vi "XY Graph.vi"() -> ()   [LabVIEW 2023]
uses:
  <vilib>/Utility/file.llb/Read Delimited Spreadsheet (DBL).vi
panel:
  out "XY Graph 3":cluster{dbl[], "all rows":dbl[]}[](graph)
  out "y":dbl[](array[numeric])
  out "x":dbl[](array[numeric])=[1.0, 2.0, 3.0, 4.0, 5.0, 6.0]
  out "XY Graph 2":cluster{dbl[], "all rows":dbl[]}(graph)
  out "y":dbl[](array[numeric])
  out "y":dbl[](array[numeric])
  in  "file path (dialog if empty)":path
  out "XY Graph":cluster{"Y":dbl[], "Y":dbl[]}[](graph)
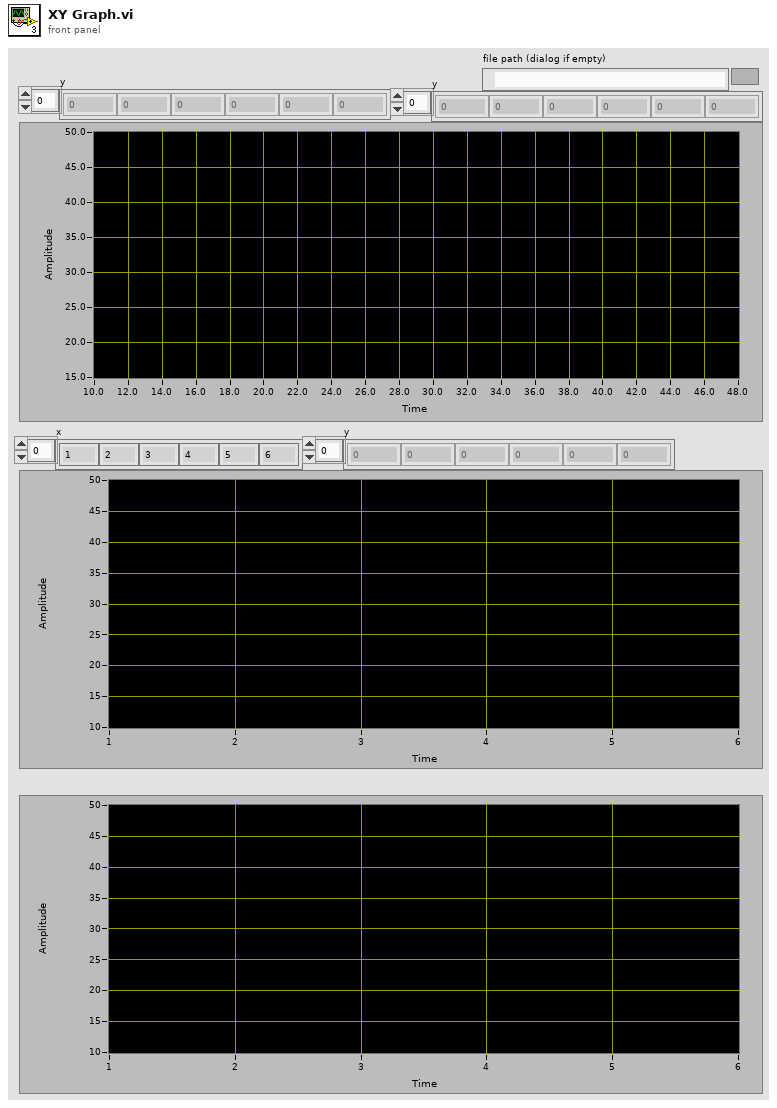
[diagram p1: front panel]
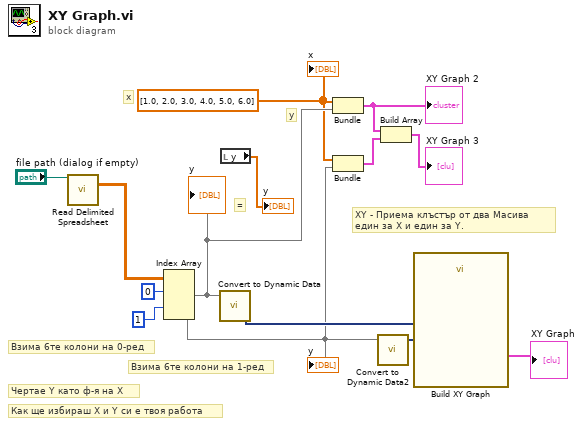
[diagram p0: block diagram]
diagram:
  w6 = dbl[] [1.0, 2.0, 3.0, 4.0, 5.0, 6.0]
  # "Как ще избираш X и Y си е твоя работа"
  # "Чертае Y като ф-я на Х"
  # "XY - Приема клъстър от два Масива\nедин за Х и един за Y."
  # "Взима 6те колони на 1-ред"
  # "Взима 6те колони на 0-ред"
  # "="
  # "y"
  # "x"
  n1 = call-poly <vilib>:"Read Delimited Spreadsheet.vi"("file path (dialog if empty)"="file path (dialog if empty)") -> ("all rows"=w12:dbl[][])  [unwired: 9 in, 5 out]
  n2 = Index Array(array=w12, index (row) #1=0 ("index (row)"), index (row) #2=1 ("index (row)")) -> (element #1=w7:dbl[], element #2=w5:dbl[])  [unwired: 2 in]
  "y" <- w7
  "y" <- w5
  n3 = call "Convert to Dynamic Data"("Array"=w7) -> ("Dynamic Data Type"=w10:dynamicdata)  [unwired: 3 in]
  n4 = local read "y"() -> (→"y":dbl[])
  n5 = Bundle(w6, "all rows"=w7) -> (w3:cluster{dbl[], "all rows":dbl[]})  [unwired: 1 in]
  "XY Graph 2" <- w3
  n6 = Bundle(w6, "all rows"=w5) -> (w4:cluster{dbl[], "all rows":dbl[]})  [unwired: 1 in]
  n7 = call "Convert to Dynamic Data2"("Array"=w5) -> ("Dynamic Data Type"=w8:dynamicdata)  [unwired: 3 in]
  n8 = Build Array(w3, w4) -> (→"XY Graph 3":cluster{dbl[], "all rows":dbl[]}[])
  n9 = call "Build XY Graph"("Y Input"=w8, "X Input"=w10) -> ("XY Graph"=→"XY Graph":cluster{"X":dbl[], "Y":dbl[]}[])  [unwired: 8 in, 1 out]
  "x" <- w6
